vi "OpenAllNodes.vi"() -> (2 "Nodes":string[][](array[string]))   [LabVIEW 2013]
uses:
  SubVIs/_ROSControl.ctl
  SubVIs/_ROSDirection.ctl
  _ROSDefinition.vi
panel:
  out "size(s)":i32
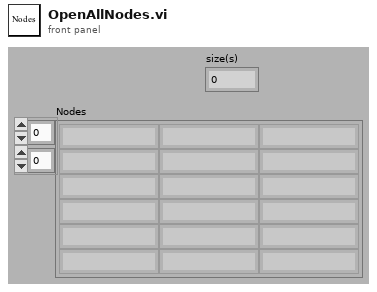
[diagram p1: front panel]
types:
  T1 = typedef "_ROSControl.ctl" = cluster{"topic port":u16, "Node":string, "topic":string, "type":string, "node port":u32, "error ":errorcluster, "Direction":T2, "APIs":string[]}
  T2 = typedef "_ROSDirection.ctl" = enum16{"Node", "Publisher", "Subscriber", "Service Client"}
  T3 = cluster{"server vi":string, "reference":refnum<vi>, "Description":string[], "Connected":bool}[]
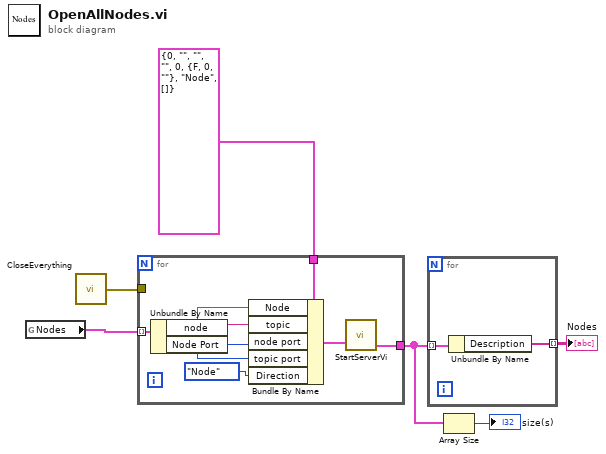
[diagram p0: block diagram]
diagram:
  n1 = global read "_ROSDefinition.vi" "Nodes"() -> (w3:cluster{"node":string, "Node Port":u32}[])
  n2 = call "CloseEverything.vi"() -> ("error out"=w5:errorcluster)  [unwired: 1 in]
  n3 = for {
    tunnel: w3 -> [w13] mode=indexing
    tunnel: T1 {"topic port"=0, "Node"="", "topic"="", "type"="", "node port"=0, "error "={"status"=FALSE, "code"=0, "source"=""}, "Direction"=enum."Node", "APIs"=[]} ("Baxter") -> [w11]
    tunnel: w5 -> [_]
    tunnel: [w7] -> w1
    n4 = Unbundle By Name(w13) -> ("node"=w9:string, "Node Port"=w8:u32)
    n5 = Bundle By Name(cluster=w11, "Node"=w9, "topic"=w9, "node port"=w8, "topic port"=w8, "Direction"=_ROSDirection."Node") -> (w12:T1)
    n6 = call "StartServerVi.vi"("Baxter"=w12) -> ("Active Topics"=w7:T3)  [unwired: 2 out]
  }
  n7 = for {
    tunnel: w1 -> [w15] mode=indexing
    tunnel: [w14] -> w4 mode=indexing
    n8 = Unbundle By Name(w15) -> ("Description"=w14:string[])
  }
  "Nodes" <- w4
  n9 = Array Size(array=w1) -> (size(s)=→"size(s)":i32)
